vi "Dashboard Main.vi"() -> ()   [LabVIEW 2013]
uses:
  <vilib>/event_ctls.llb/eventvkey.ctl
  <vilib>/Rock Robotics/WPI/Dashboard/WPI_DashboardLogging Global.vi
  <vilib>/Utility/config.llb/Write Key (String).vi
  <vilib>/Utility/config.llb/Write Key (I32).vi
  <vilib>/Utility/config.llb/NI_LVConfig.lvlib
panel:
  out "Camera Image 2":T1(plugin-control)
  out "Image Message":string="Timeout in Camera Communications"
  in  "Rec Mode":enum32{"Stop", "Record", "Playback"}(radio)
  in  "Dashboard Tab":T2(tab)
  in  "Camera Settings":T3={"Frame Rate"=30, "Compression"=30, "Size"=1} {"Frame Rate" scale=1.0..30.0; "Size" items=["640x480", "320x240", "160x120"]}
  out "MotorSliders R":cluster{"MotorSlide1":dbl, "MotorSlide2":dbl} {"MotorSlide2" scale=-1.0..1.0 scale format="%#_2e"; "MotorSlide1" scale=-1.0..1.0 scale format="%#_2e"}
  out "MotorChart R":cluster{"Numeric":dbl, "Numeric":dbl}(graph)
  out "MotorSliders L":T4 {"MotorSlide4 2" scale=0.0..14.0 scale format="%#_2e"; "MotorSlide2" scale=-1.0..1.0 scale format="%#_2e"; "MotorSlide1" scale=-1.0..1.0 scale format="%#_2e"}
  out "MotorChart L":T5(graph)
  out "JS1 Z":dbl(slide) scale=-1.0..1.0 scale format="%#_2e"
  out "Joystick 1":cluster{"X":dbl, "Y":dbl}[](graph)
  out "JS Buttons 1":T6
  out "JS2 Z":dbl(slide) scale=-1.0..1.0 scale format="%#_2e"
  out "Joystick 2":cluster{"X":dbl, "Y":dbl}[](graph)
  out "JS Buttons 2":T6
  out "Mode":T7(ring)=enum."Auto Disabled"
  out "Camera IP":string
  in  "DB Camera Config":bool
  out "fps":dbl format="%#.1g"
  out "Mbps":dbl format="%#.1g"
  out "Mbps 2":bool
  out "LED 1":bool
  out "Pressure":dbl(knob) scale=0.0..120.0
  out "Distance From Wall":dbl(knob) scale=0.0..2.0
  in  "Checkbox 2":bool
  in  "Checkbox 1":bool
  in  "Test Slider":dbl(slide) scale=0.0..100.0 scale format="%#_3g"
  in  "On/Off":bool caption="Solenoid"
  in  "Test Name":u16(ring) items=["Select the test to run...", "Example Test", "-------------------------------", "List of tests is built in robot code.", "Replace with your own automated tests."]
  in  "Test Tree":string(tree)
  in  "Motor":cluster{"Value":dbl, "Enable":bool} {"Value" scale=-1.0..1.0 scale format="%#_3g"}
  out "Progress":T8 {"Test Progress" scale=0.0..100.0}
  in  "Rev/Fwd":cluster{"Forward":bool, "Reverse":bool}
  in  "Test Ring":u16(ring) items=["Auto", "Fixed indoor", "Fixed outdoor 1", "Fixed outdoor 2", "Fixed fluorescent 1", "Fixed fluorescent 2", "Hold current"]
  in  "Listbox":i32(listbox)
  out "Tree":string(tree)
  out "Camera Image":T1(plugin-control)
  in  "Enable":bool
  # "Left"
  # "Front"
  # "Right"
  # "Battery"
  # "Customize by placing controls and indicators here and name to\nmatch Dashboard Variables on robot."
  # "This tab is a great place for autonomous settings and validation.\nCustomize by placing controls and indicators here and name to\nmatch Dashboard Variables on robot."
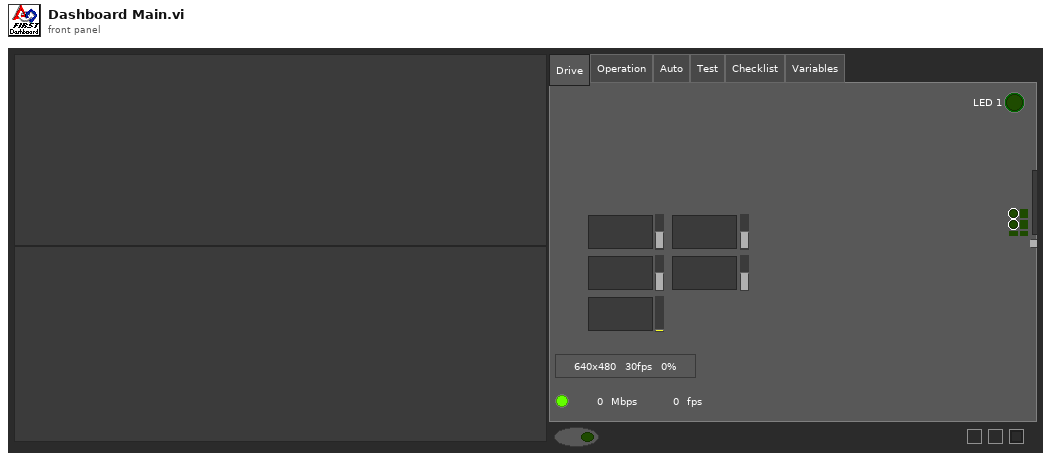
[diagram p1: front panel]
types:
  T1 = typedef "IMAQ Image.ctl" = refnum<image>
  T2 = enum32{"Drive", "Operation", "Auto", "Test", "Checklist", "Variables"}
  T3 = cluster{"Frame Rate":i32, "Compression":i32, "Size":u16}
  T4 = cluster{"MotorSlide1":dbl, "MotorSlide2":dbl, "MotorSlide4 2":dbl}
  T5 = cluster{"Numeric":dbl, "Numeric":dbl, "Battery":sgl}
  T6 = cluster{bool, bool, bool, bool, bool, bool, bool, bool, bool, bool, bool, bool}
  T7 = enum8{"Tele-Op Disabled", "Tele-Op Enabled", "Auto Disabled", "Auto Enabled", "Test Disabled", "Test Enabled", ""}
  T8 = cluster{"Test Progress":u8, "Test Progress Text":string}
  T9 = typedef "Image Type" = u32
  T10 = cluster{"Digital Inputs":bool[], "Digital Outputs":bool[]}
  T11 = cluster{"Competition mode":bool, "Robot Link":bool, "Autonomous":bool, "Enabled":bool, "E-Stop":bool, "Simulated":bool, "TestMode":bool, "Docked Window":bool}
  T12 = cluster{"Boolean Array[0]":bool, "Boolean Array[1]":bool, "Boolean Array[2]":bool, "Boolean Array[3]":bool, "Boolean Array[4]":bool, "Boolean Array[5]":bool, "Boolean Array[6]":bool, "Boolean Array[7]":bool, "Boolean Array[8]":bool, "Boolean Array[9]":bool, "Boolean Array[10]":bool, "Boolean Array[11]":bool}
  T13 = typedef "NI_LVConfig.lvlib/Config Data RefNum.ctl" = refnum<k1>
  T14 = typedef "eventvkey.ctl" = enum16{"ASCII", "Enter", "Return", "Shift", "Ctrl", "Alt", "Cmd", "Opt", "Caps", "NumLock", "Clear", "Break", "Up", "Down", "Left", "Right", "Insert", "Delete", "Home", "End", "PageUp", "PageDown", "Escape", "Help", "Pause", "ScrollLock", "F1", "F2", "F3", "F4", "F5", "F6", "F7", "F8", "F9", "F10", "F11", "F12", "F13", "F14", "F15", "F16", "F17", "F18", "F19", "F20", "F21", "F22", "F23", "F24", "Play", "VolumeUp", "VolumeDown", "Mute", "Two Byte Char"}
  T15 = cluster{"Image Size":bool, "Image Type":bool, "Pixel Value":bool, "ROI Information":bool, "Zoom Factor":bool}
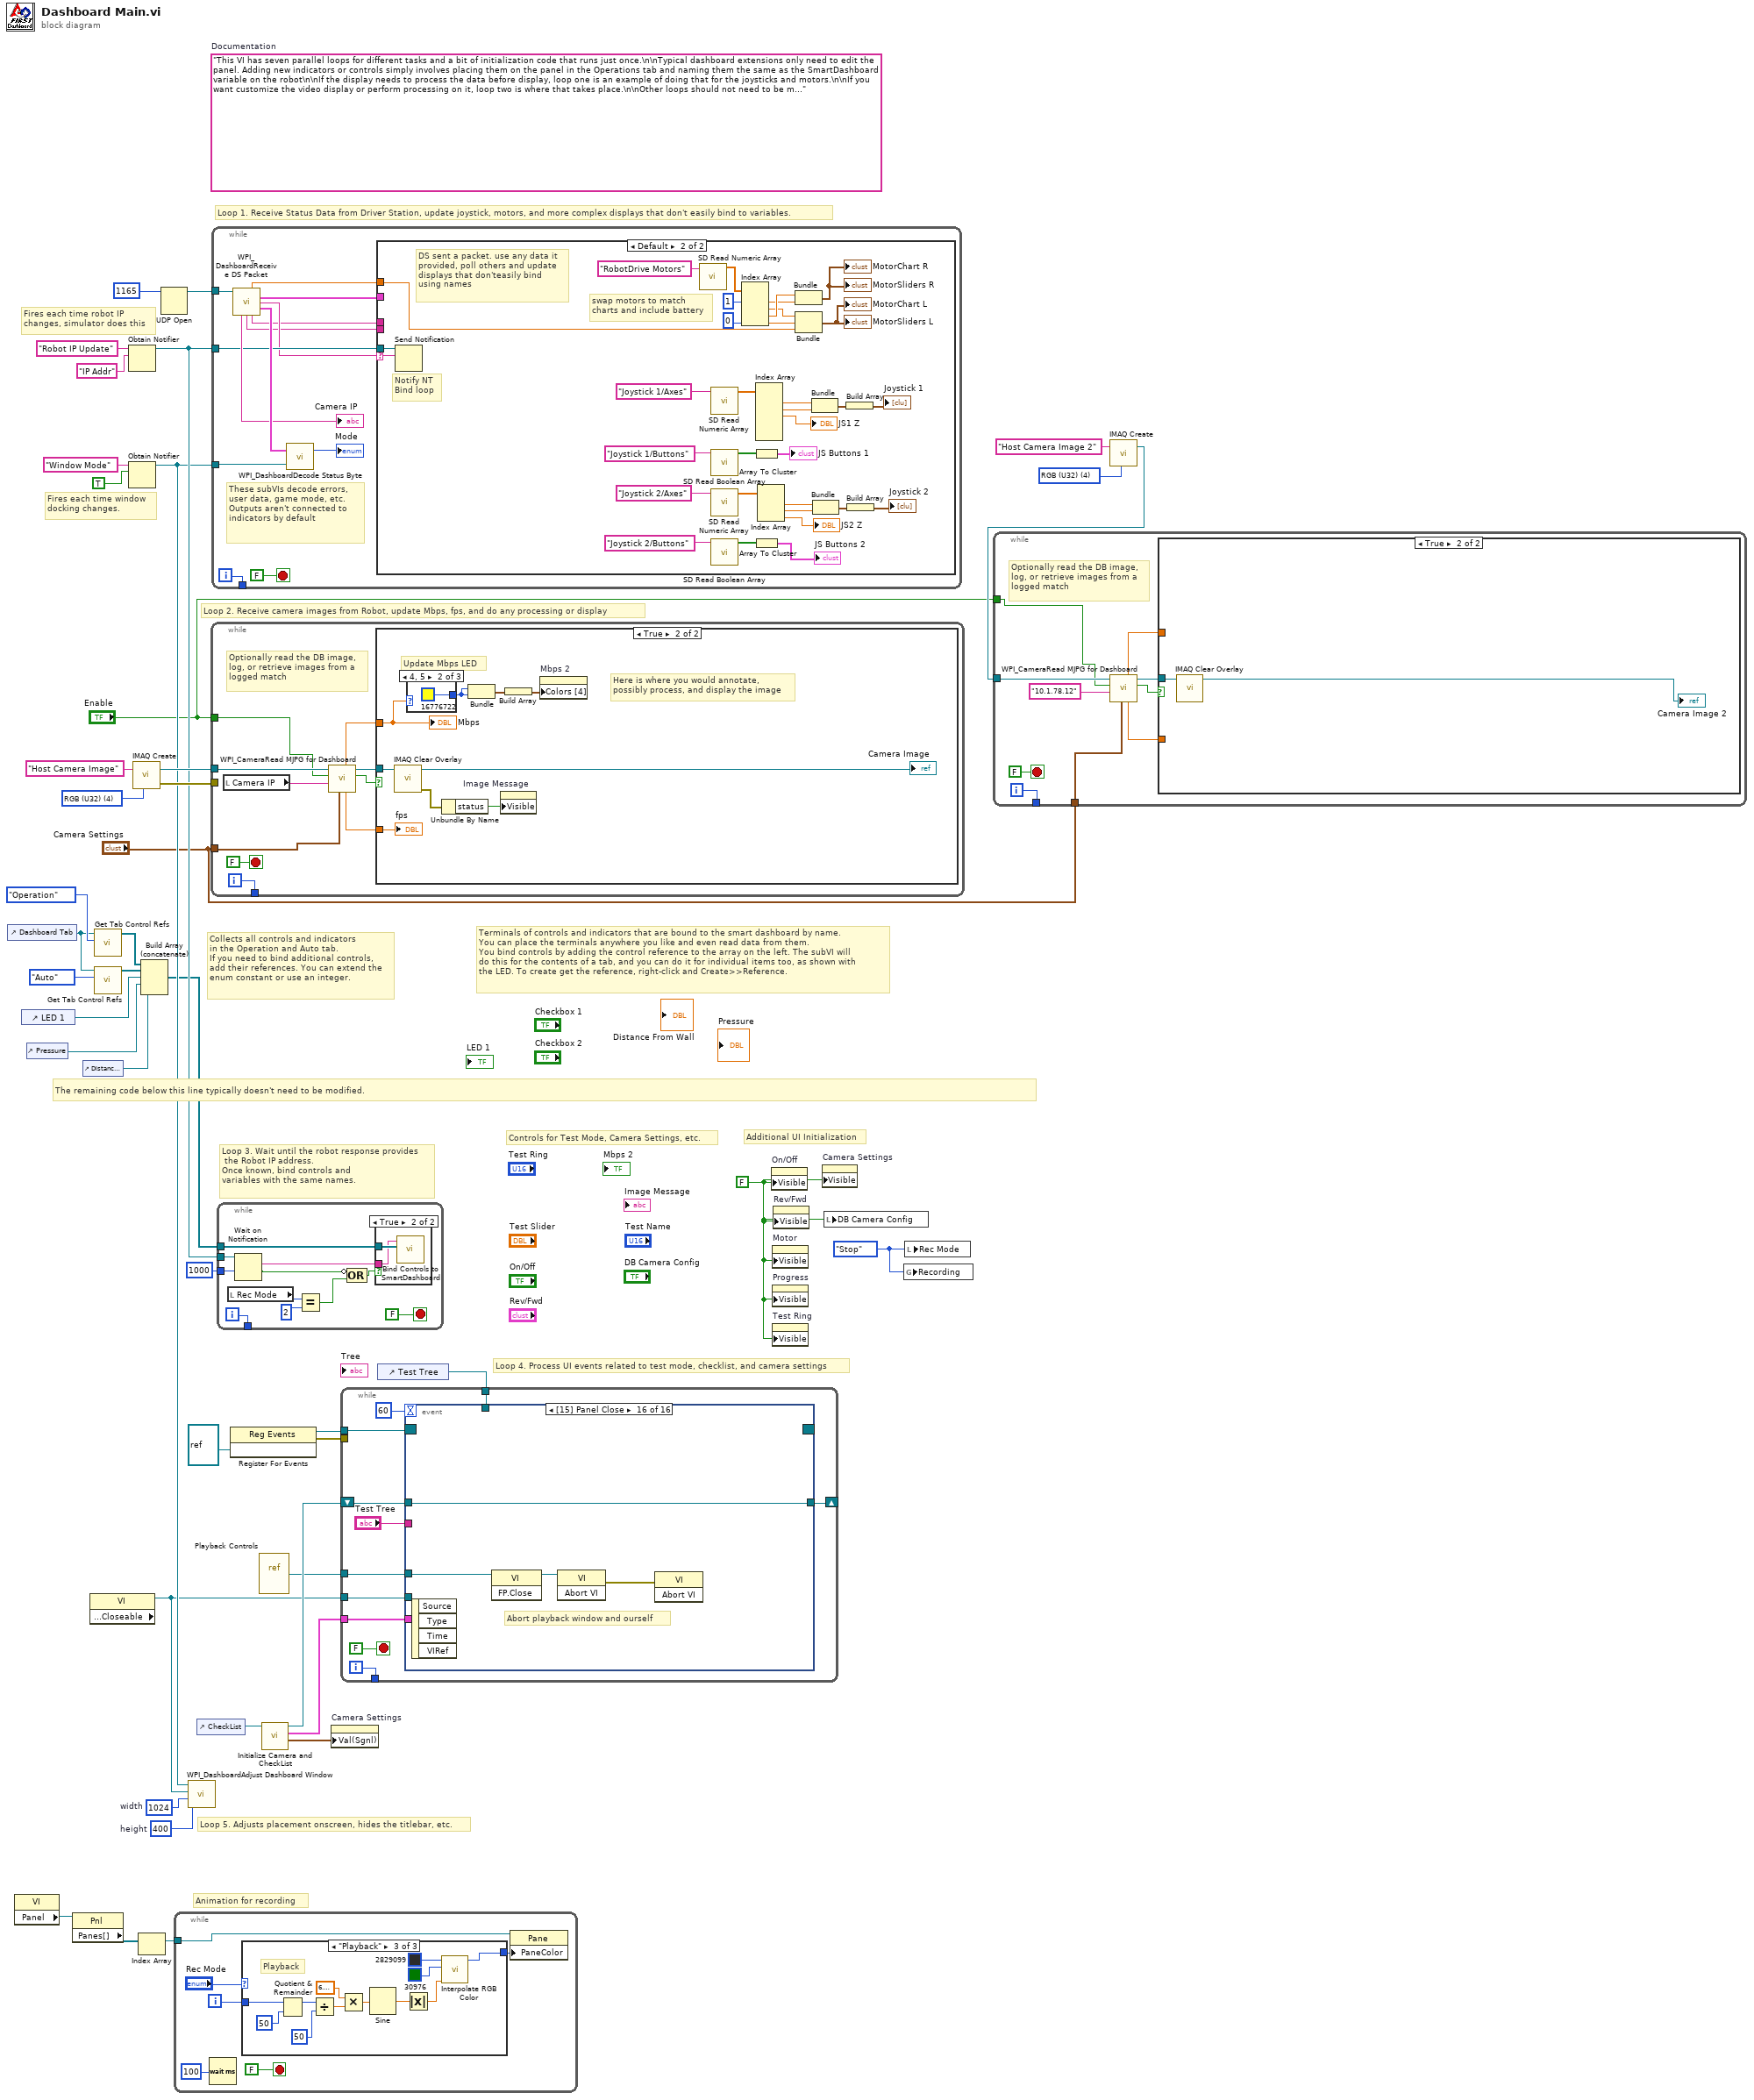
[diagram p0: block diagram]
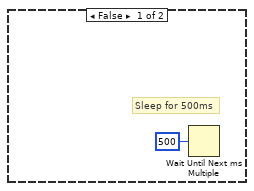
[diagram p2: hidden frame]
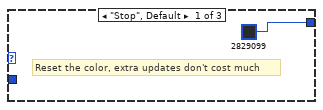
[diagram p3: hidden frame]
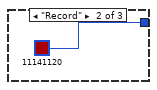
[diagram p4: hidden frame]
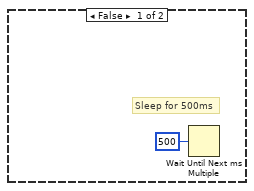
[diagram p6: hidden frame]
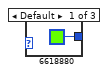
[diagram p7: hidden frame]
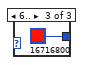
[diagram p8: hidden frame]
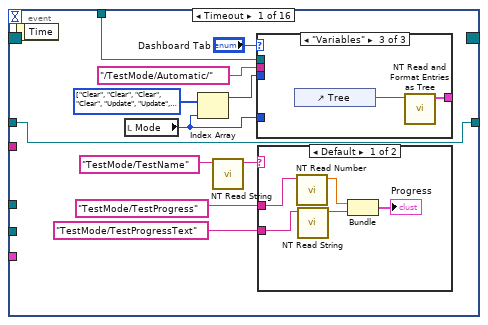
[diagram p9: hidden frame]
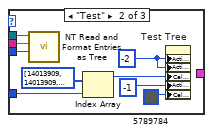
[diagram p11: hidden frame]
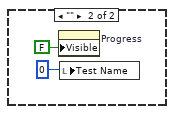
[diagram p12: hidden frame]
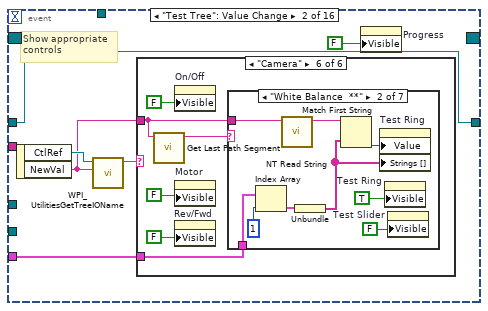
[diagram p13: hidden frame]
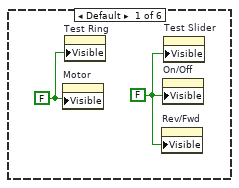
[diagram p14: hidden frame]
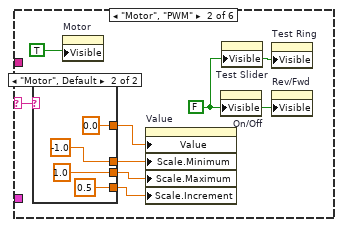
[diagram p15: hidden frame]
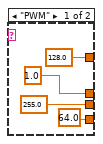
[diagram p16: hidden frame]
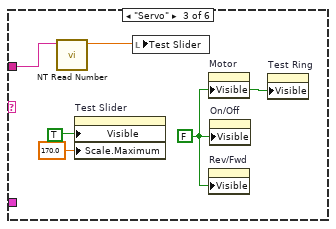
[diagram p17: hidden frame]
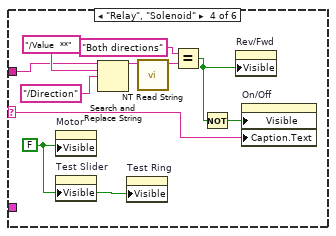
[diagram p18: hidden frame]
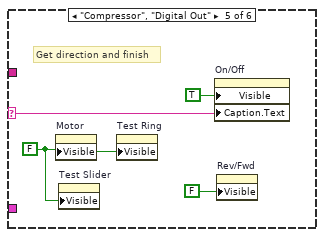
[diagram p19: hidden frame]
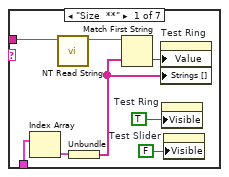
[diagram p20: hidden frame]
diagram:
  w5 = T9 4 items=["Grayscale (U8)", "Grayscale (I16)", "Grayscale (SGL)", "Complex (CSG)", "RGB (U32)", "HSL (U32)", "RGB (U64)"] ("Image Type")
  w15 = enum32{"Stop", "Record", "Playback"}."Stop" ("Rec Mode")
  w18 = 400  # height
  w19 = 1024  # width
  w32 = FALSE ("Visible")
  (unwired) "This VI has seven parallel loops for different tasks and a bit of initialization code that runs just once.\n\nTypical dashboard extensions only need to edit the panel. Adding new indicators or controls simply involves placing them on the panel in the Operations tab and naming them the same as the SmartDashboard variable on the robot\n\nIf the display needs to process the data before display, loop one is an example of doing that for the joysticks and motors.\n\nIf you want customize the video display or perform processing on it, loop two is where that takes place.\n\nOther loops should not need to be modified. They are pretty standard, and document the task they perform."  # Documentation
  w42 = T9 4 items=["Grayscale (U8)", "Grayscale (I16)", "Grayscale (SGL)", "Complex (CSG)", "RGB (U32)", "HSL (U32)", "RGB (U64)"] ("Image Type")
  # "Controls for Test Mode, Camera Settings, etc."
  # "Additional UI Initialization"
  # "Animation for recording"
  # "Fires each time robot IP\nchanges, simulator does this"
  # "Fires each time window\ndocking changes."
  # "Collects all controls and indicators\nin the Operation and Auto tab.\nIf you need to bind additional controls,\nadd their references. You can extend the\nenum constant or use an integer."
  # "The remaining code below this line typically doesn't need to be modified."
  # "Loop 4. Process UI events related to test mode, checklist, and camera settings"
  # "Terminals of controls and indicators that are bound to the smart dashboard by name.\nYou can place the terminals anywhere you like and even read data from them.\nYou bind controls by adding the control reference to the array on the left. The subVI will\ndo this for the contents of a tab, and you can do it for individual items too, as shown with\nthe LED. To create get the reference, right-click and Create>>Reference."
  # "Loop 3. Wait until the robot response provides\n the Robot IP address.\nOnce known, bind controls and\nvariables with the same names."
  # "Loop 5. Adjusts placement onscreen, hides the titlebar, etc."
  # "Loop 1. Receive Status Data from Driver Station, update joystick, motors, and more complex displays that don't easily bind to variables."
  # "Loop 2. Receive camera images from Robot, update Mbps, fps, and do any processing or display"
  n1 = control-ref of="Dashboard Tab"() -> (w13:refnum<vi>)
  n2 = property class="VI"() -> ("Panel"=w26:refnum<vi>)  [unwired: 2 in, 2 out]
  n3 = control-ref of="LED 1"() -> (w8:refnum<vi>)
  n4 = control-ref of="Pressure"() -> (w7:refnum<vi>)
  n5 = property class="Pnl"(reference=w26) -> ("Panes[]"=w27:refnum<vi>[])  [unwired: 1 in, 2 out]
  n6 = control-ref of="Distance From Wall"() -> (w6:refnum<vi>)
  n7 = property class="VI" props=["Front Panel.Closeable"]() -> (reference out=w14:refnum<vi>)  [unwired: 2 in, 2 out]
  n8 = call <vilib>:"Get Tab Control Refs.vi"("Page Index"=T2."Operation" ("Dashboard Tab"), "TabControl in"=w13) -> ("ControlsOnPage"=w11:refnum<vi>[])  [unwired: 9 in]
  n9 = call <vilib>:"Get Tab Control Refs.vi"("Page Index"=T2."Auto" ("Dashboard Tab"), "TabControl in"=w13) -> ("ControlsOnPage"=w12:refnum<vi>[])  [unwired: 9 in]
  n10 = Obtain Notifier(name (unnamed)="Robot IP Update", notification data type="IP Addr" ("name (unnamed)")) -> (notifier out=w36:refnum<notifier>)  [unwired: 2 in, 2 out]
  n11 = Obtain Notifier(name (unnamed)="Window Mode", notification data type=TRUE) -> (notifier out=w17:refnum<notifier>)  [unwired: 2 in, 2 out]
  n12 = call "IMAQ Create"("Image Name"="Host Camera Image", "Image Type"=w42) -> ("New Image"=w40:T1, "error out"=w39:errorcluster)  [unwired: 2 in, 1 out]
  n13 = Index Array(array=w27) -> (element=w25:refnum<vi>)  [unwired: 1 in]
  n14 = Build Array (concatenate)(w11, w12, w8, w7, w6) -> (w10:refnum<vi>[])
  n15 = UDP Open(11:u16 1165 ("port")) -> (port=w43:refnum<k16>)  [unwired: 2 in, 4 out]
  n16 = while {
    tunnel: w25 -> [w46]
    i -> [w49]
    stop <- FALSE stop-if-true
    n17 = Wait (ms)(milliseconds to wait=u32 100) -> ()  [unwired: 1 out]
    n18 = case shown="\"Playback\"" "Rec Mode" {
      tunnel: w49 -> [_ _ w64]
      tunnel: [u32 2829099 ("Base Color") u32 11141120 ("Target Color") w53] -> w45
      frame "Stop", Default {
        # "Reset the color, extra updates don't cost much"
      }
      frame "Record" {
      }
      frame "Playback" {
        # "Playback"
        n19 = Quotient & Remainder(x=w64, y=u32 50 ("milliseconds to wait")) -> (x-y*floor(x/y)=w60:u32)  [unwired: 1 out]
        n20 = Divide(x=w60, y=u32 50 ("milliseconds to wait")) -> (x/y=w57:dbl)
        n21 = Multiply(x=6.283185307179586, y=w57) -> (x*y=w62:dbl)
        n22 = Sine(x=w62) -> (sin(x)=w61:dbl)
        n23 = Absolute Value(x=w61) -> (abs(x)=w54:dbl)
        n24 = call "Interpolate RGB Color.vi"("Proportion"=w54, "Target Color"=u32 30976, "Base Color"=u32 2829099) -> ("Result Color"=w53:u32)  [unwired: 8 in]
      }
    }
    n25 = property class="Pane"(reference=w46, "PaneColor"=w45) -> ()  [unwired: 1 in, 2 out]
  }
  n26 = call <vilib>:"WPI_DashboardAdjust Dashboard Window.vi"("height"=w18, "width"=w19, "reference in"=w14, "Notifier in"=w17) -> ()  [unwired: 8 in]
  n27 = control-ref of="CheckList"() -> (w16:refnum<vi>)
  n28 = while {
    tunnel: w40 -> [w72]
    tunnel: w39 -> [_]
    tunnel: [w73] -> _
    tunnel: "Camera Settings" -> [w66]
    tunnel: "Enable" -> [w65]
    i -> [w73]
    stop <- FALSE stop-if-true
    # "Optionally read the DB image,\nlog, or retrieve images from a\nlogged match"
    n29 = local read "Camera IP"() -> (w67:string)
    n30 = call <vilib>:"WPI_CameraRead MJPG for Dashboard.vi"("Camera Settings"=w66, "Camera IP"=w67, "Enable"=w65, "Refnum in"=w72) -> ("Active"=w70:bool, "Refnum out"=w71:T1, "FPS"=w69:dbl, "Bandwidth (Mbps)"=w68:dbl)  [unwired: 4 in]
    n31 = case shown="True" w70 {
      tunnel: w71 -> [_ w79]
      tunnel: w68 -> [_ w78]
      tunnel: w69 -> [_ w76]
      frame False {
        # "Sleep for 500ms"
        n32 = Wait Until Next ms Multiple(millisecond multiple=u32 500) -> ()  [unwired: 1 out]
      }
      frame True {
        # "Here is where you would annotate,\npossibly process, and display the image"
        # "Update Mbps LED"
        n33 = call "IMAQ Clear Overlay"("Image"=w79) -> ("error out"=w83:errorcluster, "Image Out"=→"Camera Image":T1)  [unwired: 2 in, 7 out]
        n34 = case shown="4, 5" w78 {
          tunnel: [u32 6618880 ("Color Box") u32 16776722 ("Color Box") u32 16716800 ("Color Box")] -> w80
          frame Default {
          }
          frame 4, 5 {
          }
          frame 6.. {
          }
        }
        n35 = Unbundle By Name(w83) -> ("status"=w84:bool)
        n36 = Bundle("Color Box"=w80, "Color Box"=w80) -> (w82:cluster{"Color Box":u32, "Color Box":u32})  [unwired: 1 out]
        n37 = property on="Image Message" class="Str"("Visible"=w84) -> ()  [unwired: 2 in, 2 out]
        n38 = Build Array(w82) -> (w81:cluster{"Color Box":u32, "Color Box":u32}[])
        n39 = property on="Mbps 2" class="Bool (strict)"("Colors [4]"=w81) -> ()  [unwired: 2 in, 2 out]
        "Mbps" <- w78
        "fps" <- w76
      }
    }
  }
  n40 = while {
    tunnel: w43 -> [w98]
    tunnel: w36 -> [w93]
    tunnel: w17 -> [w97]
    tunnel: [w94] -> _
    i -> [w94]
    stop <- FALSE stop-if-true
    # "These subVIs decode errors, user data, game mode, etc.\nOutputs aren't connected to indicators by default"
    n41 = call <vilib>:"WPI_DashboardReceive DS Packet.vi"("Recv Socket"=w98) -> ("Battery"=w88:sgl, "Driver Station"=w89:T10, "Robot IP Address"=w92:string, "Status"=w99:T11, "Camera IP Address"=→"Camera IP":string, "Low Priority User Data"=w91:string, "High Priority User Data"=w90:string)  [unwired: 1 in, 7 out]
    n42 = call <vilib>:"WPI_DashboardDecode Status Byte.vi"("Window Mode Notifier"=w97, "Status"=w99) -> ("Mode"=→"Mode":T7)  [unwired: 1 out]
    n43 = case shown="Default" w92 {
      selector: w92 -> [_ w111]
      tunnel: w93 -> [_ w112]
      tunnel: w91 -> [_ _]
      tunnel: w90 -> [_ _]
      tunnel: w89 -> [_ _]
      tunnel: w88 -> [_ w110]
      frame "0.0.0.0" {
        # "DS not sending packets, or no robot exists yet.\nDon't poll the variables"
      }
      frame Default {
        # "Notify NT\nBind loop"
        # "DS sent a packet. use any data it\nprovided, poll others and update\ndisplays that don'teasily bind\nusing names"
        # "swap motors to match\ncharts and include battery"
        n44 = Send Notification(notification=w111, notifier=w112) -> ()  [unwired: 1 in, 2 out]
        n45 = call <vilib>:"SD Read Numeric Array.vi"("Name"="RobotDrive Motors") -> ("Numeric Array"=w109:dbl[])  [unwired: 8 in, 2 out]
        n46 = call <vilib>:"SD Read Numeric Array.vi"("Name"="Joystick 1/Axes") -> ("Numeric Array"=w128:dbl[])  [unwired: 8 in, 2 out]
        n47 = call <vilib>:"SD Read Boolean Array.vi"("Name"="Joystick 1/Buttons") -> ("Boolean Array"=w130:bool[])  [unwired: 8 in, 2 out]
        n48 = call <vilib>:"SD Read Numeric Array.vi"("Name"="Joystick 2/Axes") -> ("Numeric Array"=w122:dbl[])  [unwired: 8 in, 2 out]
        n49 = call <vilib>:"SD Read Boolean Array.vi"("Name"="Joystick 2/Buttons") -> ("Boolean Array"=w121:bool[])  [unwired: 8 in, 2 out]
        n50 = Index Array(array=w109, index #1=1, index #4=0) -> (element #1=w105:dbl, element #2=w104:dbl, element #3=w106:dbl, element #4=w101:dbl)  [unwired: 2 in]
        n51 = Array To Cluster(array=w130) -> (cluster=→"JS Buttons 1":T12)
        n52 = Array To Cluster(array=w121) -> (cluster=→"JS Buttons 2":T12)
        n53 = Index Array(array=w128) -> (element #1=w125:dbl, element #2=w126:dbl, element #3=→"JS1 Z":dbl)  [unwired: 6 in, 3 out]
        n54 = Index Array(array=w122) -> (element #1=w117:dbl, element #2=w116:dbl, element #3=→"JS2 Z":dbl)  [unwired: 3 in]
        n55 = Bundle("Numeric"=w106, "Numeric"=w105) -> (→"MotorChart R" →"MotorSliders R":cluster{"Numeric":dbl, "Numeric":dbl})  [unwired: 1 in]
        n56 = Bundle("Numeric"=w104, "Numeric"=w101, "Battery"=w110) -> (→"MotorChart L" →"MotorSliders L":T5)  [unwired: 1 in]
        n57 = Bundle("Numeric"=w125, "Numeric"=w126) -> (w124:cluster{"Numeric":dbl, "Numeric":dbl})  [unwired: 1 in]
        n58 = Bundle("Numeric"=w117, "Numeric"=w116) -> (w118:cluster{"Numeric":dbl, "Numeric":dbl})  [unwired: 1 in]
        n59 = Build Array(w124) -> (→"Joystick 1":cluster{"Numeric":dbl, "Numeric":dbl}[])
        n60 = Build Array(w118) -> (→"Joystick 2":cluster{"Numeric":dbl, "Numeric":dbl}[])
      }
    }
  }
  n61 = while {
    tunnel: w10 -> [w144]
    tunnel: w36 -> [w142]
    tunnel: [w140] -> _
    tunnel: u32 1000 ("milliseconds to wait") -> [w139]
    i -> [w140]
    stop <- FALSE stop-if-true
    n62 = local read "Rec Mode"() -> (w135:enum32{"Stop", "Record", "Playback"})
    n63 = Wait on Notification(notifier=w142, timeout in ms (-1)=w139) -> (notification=w141:string, timed out?=w137:bool)  [unwired: 2 in, 2 out]
    n64 = Equal?(x=w135, y=u16 2 ("Rec Mode")) -> (x = y?=w136:bool)
    n65 = Compound Arithmetic op=OR(invert w137, w136) -> (w138:bool)
    n66 = case shown="True" w138 {
      tunnel: w144 -> [_ w146]
      tunnel: w141 -> [_ w145]
      frame False {
      }
      frame True {
        n67 = call <vilib>:"Bind Controls to SmartDashboard.vi"("Bound Control Refs"=w146, "Server IP Address"=w145) -> ()  [unwired: 10 in]
      }
    }
  }
  n68 = register-events(refnum<vi> refnum) -> (reference out=w23:refnum<event-registration>, error out=w22:errorcluster)  [unwired: 2 in]
  n69 = vi-ref "Playback Controls.vi"() -> (w24:refnum<vi>)
  n70 = call "Initialize Camera and CheckList.vi"("ListBox in"=w16) -> ("Cluster"=w30:cluster{"value":i32, "value":i32, "index":i32}, "Array"=w31:cluster{string[]}[], "File Refnum"=w29:T13)  [unwired: 8 in]
  n71 = property on="Camera Settings" class="Clust (strict)"("Val(Sgnl)"=w30) -> ()  [unwired: 2 in, 2 out]
  n72 = control-ref of="Test Tree"() -> (w28:refnum<vi>)
  n73 = while {
    tunnel: w31 -> [w154]
    shift-right: [w153] -> _
    shift-left: w29 -> [w152]
    tunnel: [w151] -> _
    tunnel: w28 -> [w150]
    tunnel: w24 -> [w149]
    tunnel: w23 -> [w148]
    tunnel: w22 -> [_]
    tunnel: w14 -> [w147]
    i -> [w151]
    stop <- FALSE stop-if-true
    n74 = event shown="[15] Panel Close" {
      selector: w148 -> [_ _ _ _ _ _ _ _ _ _ _ _ _ _ _ _]
      dyn-events: [_ _ _ _ _ _ _ _ _ _ _ _ _ w392 _ _] -> _
      timeout: u32 60 ("milliseconds to wait") -> [_ _ _ _ _ _ _ _ _ _ _ _ _ _ _ _]
      tunnel: w150 -> [w164 _ _ _ _ _ _ _ _ _ _ _ _ _ _ _]
      tunnel: "Test Tree" -> [_ _ _ _ _ _ _ _ w361 w369 w371 w375 w383 _ _ _]
      tunnel: w154 -> [_ w188 _ _ _ _ w325 w355 _ _ _ _ _ _ _ _]
      tunnel: [w158 w187 w286 w291 w299 w311 w324 w348 w360 w367 w370 w374 w382 w394 w408 w409] -> w153
      tunnel: w152 -> [w158 w187 w286 w291 w299 w311 w323 w348 w360 w367 w370 w374 w382 w394 w408 w409]
      tunnel: w149 -> [_ _ _ _ _ _ _ _ _ _ _ _ _ w395 _ w412]
      tunnel: w147 -> [_ _ _ _ _ _ _ _ _ _ _ _ _ w390 _ _]
      event Timeout {
        w163 = enum16{"Update", "Clear"}[] [enum."Clear", enum."Clear", enum."Clear", enum."Clear", enum."Update", enum."Update", enum."Clear"] items=["Update", "Clear"]
        n75 = event-data() -> ()  [unwired: 1 in, 1 out]
        n76 = local read "Mode"() -> (w161:T7)
        n77 = Index Array(array=w163, index=w161) -> (element=w162:enum16{"Update", "Clear"})
        n78 = call <vilib>:"NT Read String.vi"("Name"="TestMode/TestName") -> ("String"=w167:string)  [unwired: 9 in, 1 out]
        n79 = case shown="\"Variables\"" "Dashboard Tab" {
          tunnel: w164 -> [_ w177 _]
          tunnel: "/TestMode/Automatic/" ("Name Pattern") -> [_ w176 _]
          tunnel: w162 -> [_ w175 _]
          tunnel: w161 -> [_ w173 _]
          tunnel: [_ _ w179] -> _
          frame "Operation", Default {
          }
          frame "Test" {
            w172 = -2 ("Active Item:Row Number")
            n80 = call <vilib>:"NT Read and Format Entries as Tree.vi"("Operation"=w175, "Name Pattern"=w176, "Tree Refnum"=w177) -> ()  [unwired: 7 in, 2 out]
            n81 = Index Array(array=u32[] [14013909, 14013909, 14013909, 14013909, 14013909, 16777215, 14013909], index=w173) -> (element=w171:u32)
            n82 = property on="Test Tree" class="Tree (strict)"("Active Item Row Number"=w172, "ActiveColNum"=w172, "CellBG"=w171, "Active Item Row Number"=-1 ("Active Item:Row Number"), "CellBG"=u32 5789784 ("Color Box")) -> ()  [unwired: 2 in, 2 out]
          }
          frame "Variables" {
            n83 = control-ref of="Tree"() -> (w178:refnum<vi>)
            n84 = call <vilib>:"NT Read and Format Entries as Tree.vi"("Tree Refnum"=w178) -> ("Formatted Strings"=w179:cluster{"Name":string, "Value":string}[])  [unwired: 9 in, 1 out]
          }
        }
        n85 = case shown="Default" w167 {
          tunnel: "TestMode/TestProgress" ("Name") -> [w181 _]
          tunnel: "TestMode/TestProgressText" ("Name") -> [w180 _]
          frame Default {
            n86 = call <vilib>:"NT Read Number.vi"("Name"=w181) -> ("Numeric"=w182:dbl)  [unwired: 9 in, 1 out]
            n87 = call <vilib>:"NT Read String.vi"("Name"=w180) -> ("String"=w183:string)  [unwired: 9 in, 1 out]
            n88 = Bundle("Numeric"=w182, "String"=w183) -> (→"Progress":cluster{"Numeric":dbl, "String":string})  [unwired: 1 in]
          }
          frame "" {
            n89 = property on="Progress" class="Clust (strict)"("Visible"=FALSE) -> ()  [unwired: 2 in, 2 out]
            n90 = local write "Test Name"(u16 0) -> ()
          }
        }
      }
      event "Test Tree": Value Change {
        # "Show appropriate\ncontrols"
        n91 = event-data() -> ("CtlRef"=w191:refnum<vi>, "NewVal"=w189:string)  [unwired: 1 in]
        n92 = call <vilib>:"WPI_UtilitiesGetTreeIOName.vi"("NewVal"=w189, "TreeControl in"=w191) -> ("I/O Name"=w192:string)  [unwired: 9 in]
        n93 = case shown="\"Camera\"" w192 {
          selector: w192 -> [_ w199 _ w217 w226 _]
          tunnel: w189 -> [_ _ w214 w216 _ w233]
          tunnel: w188 -> [_ _ _ _ _ w232]
          frame Default {
            w194 = FALSE ("Visible")
            w193 = FALSE ("Visible")
            n94 = property on="Motor" class="Clust (strict)"("Visible"=w193) -> ()  [unwired: 2 in, 2 out]
            n95 = property on="Test Ring" class="Ring (strict)"("Visible"=w193) -> ()  [unwired: 2 in, 2 out]
            n96 = property on="Rev/Fwd" class="Clust (strict)"("Visible"=w194) -> ()  [unwired: 2 in, 2 out]
            n97 = property on="On/Off" class="Bool (strict)"("Visible"=w194) -> ()  [unwired: 2 in, 2 out]
            n98 = property on="Test Slider" class="Slide (strict)"("Visible"=w194) -> ()  [unwired: 2 in, 2 out]
          }
          frame "Motor", "PWM" {
            w200 = FALSE ("Visible")
            n99 = case shown="\"Motor\", Default" w199 {
              tunnel: [1.0 ("Value") -1.0 ("Value")] -> w198
              tunnel: [255.0 ("Value") 1.0 ("Value")] -> w197
              tunnel: [128.0 ("Value") 0.0 ("Value")] -> w196
              tunnel: [64.0 ("Value") 0.5 ("Value")] -> w195
              frame "PWM" {
              }
              frame "Motor", Default {
              }
            }
            n100 = property on="Motor" class="Clust (strict)"("Visible"=TRUE) -> ()  [unwired: 2 in, 2 out]
            n101 = property on="Value" class="Slide (strict)"("Value"=w196, "Scale.Minimum"=w198, "Scale.Maximum"=w197, "Scale.Increment"=w195) -> ()  [unwired: 2 in, 2 out]
            n102 = property on="On/Off" class="Bool (strict)"("Visible"=w200) -> ()  [unwired: 2 in, 2 out]
            n103 = property on="Test Slider" class="Slide (strict)"("Visible"=w200) -> ()  [unwired: 2 in, 2 out]
            n104 = property on="Test Ring" class="Ring (strict)"("Visible"=w200) -> ()  [unwired: 2 in, 2 out]
            n105 = property on="Rev/Fwd" class="Clust (strict)"("Visible"=w200) -> ()  [unwired: 2 in, 2 out]
          }
          frame "Servo" {
            w212 = FALSE ("Visible")
            n106 = call <vilib>:"NT Read Number.vi"("Name"=w214) -> ("Numeric"=w213:dbl)  [unwired: 9 in, 1 out]
            n107 = property on="Test Slider" class="Slide (strict)"("Visible"=TRUE, "Scale.Maximum"=170.0 ("Scale.Range:Maximum")) -> ()  [unwired: 2 in, 2 out]
            n108 = local write "Test Slider"(w213) -> ()
            n109 = property on="Motor" class="Clust (strict)"("Visible"=w212) -> ()  [unwired: 2 in, 2 out]
            n110 = property on="Rev/Fwd" class="Clust (strict)"("Visible"=w212) -> ()  [unwired: 2 in, 2 out]
            n111 = property on="On/Off" class="Bool (strict)"("Visible"=w212) -> ()  [unwired: 2 in, 2 out]
            n112 = property on="Test Ring" class="Ring (strict)"("Visible"=w212) -> ()  [unwired: 2 in, 2 out]
          }
          frame "Relay", "Solenoid" {
            w215 = FALSE ("Visible")
            n113 = property on="Motor" class="Clust (strict)"("Visible"=w215) -> ()  [unwired: 2 in, 2 out]
            n114 = property on="Test Slider" class="Slide (strict)"("Visible"=w215) -> ()  [unwired: 2 in, 2 out]
            n115 = Search and Replace String(input string=w216, search string="/Value  **", replace string="/Direction") -> (result string=w222:string)  [unwired: 5 in, 3 out]
            n116 = property on="Test Ring" class="Ring (strict)"("Visible"=w215) -> ()  [unwired: 2 in, 2 out]
            n117 = call <vilib>:"NT Read String.vi"("Name"=w222) -> ("String"=w220:string)  [unwired: 9 in, 1 out]
            n118 = Equal?(x="Both directions", y=w220) -> (x = y?=w218:bool)
            n119 = Not(x=w218) -> (.not. x?=w219:bool)
            n120 = property on="Rev/Fwd" class="Clust (strict)"("Visible"=w218) -> ()  [unwired: 2 in, 2 out]
            n121 = property on="On/Off" class="Bool (strict)"("Visible"=w219, "Caption.Text"=w217) -> ()  [unwired: 2 in, 2 out]
          }
          frame "Compressor", "Digital Out" {
            w225 = FALSE ("Visible")
            # "Get direction and finish"
            n122 = property on="Motor" class="Clust (strict)"("Visible"=w225) -> ()  [unwired: 2 in, 2 out]
            n123 = property on="Test Slider" class="Slide (strict)"("Visible"=w225) -> ()  [unwired: 2 in, 2 out]
            n124 = property on="Test Ring" class="Ring (strict)"("Visible"=w225) -> ()  [unwired: 2 in, 2 out]
            n125 = property on="On/Off" class="Bool (strict)"("Visible"=TRUE, "Caption.Text"=w226) -> ()  [unwired: 2 in, 2 out]
            n126 = property on="Rev/Fwd" class="Clust (strict)"("Visible"=FALSE) -> ()  [unwired: 2 in, 2 out]
          }
          frame "Camera" {
            n127 = call <vilib>:"Get Last Path Segment.vi"("String in"=w233) -> ("String out"=w234:string)  [unwired: 10 in]
            n128 = property on="On/Off" class="Bool (strict)"("Visible"=FALSE) -> ()  [unwired: 2 in, 2 out]
            n129 = property on="Motor" class="Clust (strict)"("Visible"=FALSE) -> ()  [unwired: 2 in, 2 out]
            n130 = property on="Rev/Fwd" class="Clust (strict)"("Visible"=FALSE) -> ()  [unwired: 2 in, 2 out]
            n131 = case shown="\"White Balance  **\"" w234 {
              tunnel: w233 -> [w240 w249 w258 w267 w276 _ w282]
              tunnel: w232 -> [w238 w246 w255 w264 w273 _ _]
              frame "Size  **" {
                n132 = Index Array(array=w238) -> (element=w237:cluster{string[]})  [unwired: 1 in]
                n133 = call <vilib>:"NT Read String.vi"("Name"=w240) -> ("String"=w239:string)  [unwired: 9 in, 1 out]
                n134 = Unbundle(w237) -> (w235:string[])
                n135 = Match First String(2:w235, 3:w239) -> (0:w236:i32)  [unwired: 1 out]
                n136 = property on="Test Ring" class="Ring (strict)"("Value"=w236, "Strings []"=w235) -> ()  [unwired: 2 in, 2 out]
                n137 = property on="Test Ring" class="Ring (strict)"("Visible"=TRUE) -> ()  [unwired: 2 in, 2 out]
                n138 = property on="Test Slider" class="Slide (strict)"("Visible"=FALSE) -> ()  [unwired: 2 in, 2 out]
              }
              frame "White Balance  **" {
                n139 = Index Array(array=w246, index=1) -> (element=w247:cluster{string[]})
                n140 = call <vilib>:"NT Read String.vi"("Name"=w249) -> ("String"=w248:string)  [unwired: 9 in, 1 out]
                n141 = Unbundle(w247) -> (w244:string[])
                n142 = Match First String(2:w244, 3:w248) -> (0:w243:i32)  [unwired: 1 out]
                n143 = property on="Test Ring" class="Ring (strict)"("Value"=w243, "Strings []"=w244) -> ()  [unwired: 2 in, 2 out]
                n144 = property on="Test Ring" class="Ring (strict)"("Visible"=TRUE) -> ()  [unwired: 2 in, 2 out]
                n145 = property on="Test Slider" class="Slide (strict)"("Visible"=FALSE) -> ()  [unwired: 2 in, 2 out]
              }
              frame "Exposure  **" {
                n146 = Index Array(array=w255, index=2) -> (element=w256:cluster{string[]})
                n147 = call <vilib>:"NT Read String.vi"("Name"=w258) -> ("String"=w257:string)  [unwired: 9 in, 1 out]
                n148 = Unbundle(w256) -> (w252:string[])
                n149 = Match First String(2:w252, 3:w257) -> (0:w253:i32)  [unwired: 1 out]
                n150 = property on="Test Ring" class="Ring (strict)"("Value"=w253, "Strings []"=w252) -> ()  [unwired: 2 in, 2 out]
                n151 = property on="Test Ring" class="Ring (strict)"("Visible"=TRUE) -> ()  [unwired: 2 in, 2 out]
                n152 = property on="Test Slider" class="Slide (strict)"("Visible"=FALSE) -> ()  [unwired: 2 in, 2 out]
              }
              frame "Exposure Priority  **" {
                n153 = Index Array(array=w264, index=3) -> (element=w265:cluster{string[]})
                n154 = call <vilib>:"NT Read String.vi"("Name"=w267) -> ("String"=w266:string)  [unwired: 9 in, 1 out]
                n155 = Unbundle(w265) -> (w261:string[])
                n156 = Match First String(2:w261, 3:w266) -> (0:w262:i32)  [unwired: 1 out]
                n157 = property on="Test Ring" class="Ring (strict)"("Value"=w262, "Strings []"=w261) -> ()  [unwired: 2 in, 2 out]
                n158 = property on="Test Ring" class="Ring (strict)"("Visible"=TRUE) -> ()  [unwired: 2 in, 2 out]
                n159 = property on="Test Slider" class="Slide (strict)"("Visible"=FALSE) -> ()  [unwired: 2 in, 2 out]
              }
              frame "Color Enable  **" {
                n160 = Index Array(array=w273, index=4) -> (element=w274:cluster{string[]})
                n161 = call <vilib>:"NT Read String.vi"("Name"=w276) -> ("String"=w275:string)  [unwired: 9 in, 1 out]
                n162 = Unbundle(w274) -> (w270:string[])
                n163 = Match First String(2:w270, 3:w275) -> (0:w271:i32)  [unwired: 1 out]
                n164 = property on="Test Ring" class="Ring (strict)"("Value"=w271, "Strings []"=w270) -> ()  [unwired: 2 in, 2 out]
                n165 = property on="Test Ring" class="Ring (strict)"("Visible"=TRUE) -> ()  [unwired: 2 in, 2 out]
                n166 = property on="Test Slider" class="Slide (strict)"("Visible"=FALSE) -> ()  [unwired: 2 in, 2 out]
              }
              frame Default {
                n167 = property on="Test Ring" class="Ring (strict)"("Visible"=FALSE) -> ()  [unwired: 2 in, 2 out]
                n168 = property on="Test Slider" class="Slide (strict)"("Visible"=FALSE) -> ()  [unwired: 2 in, 2 out]
              }
              frame "Brightness  **", "Color Level  **", "Compression  **", "FPS  **", "Sharpness  **" {
                n169 = call <vilib>:"NT Read Number.vi"("Name"=w282) -> ("Numeric"=w281:dbl)  [unwired: 9 in, 1 out]
                n170 = local write "Test Slider"(w281) -> ()
                n171 = property on="Test Slider" class="Slide (strict)"("Visible"=TRUE, "Scale.Maximum"=100.0 ("Scale.Range:Maximum")) -> ()  [unwired: 2 in, 2 out]
                n172 = property on="Test Ring" class="Ring (strict)"("Visible"=FALSE) -> ()  [unwired: 2 in, 2 out]
              }
            }
          }
        }
        n173 = property on="Progress" class="Clust (strict)"("Visible"=FALSE) -> ()  [unwired: 2 in, 2 out]
      }
      event "Test Name": Mouse Enter {
        # "Populate the ring with the list of tests"
        n174 = event-data() -> ()  [unwired: 1 in, 1 out]
        n175 = call <vilib>:"NT Read String Array.vi"("Name"="TestMode/TestList") -> ("String Array"=w290:string[])  [unwired: 9 in, 1 out]
        n176 = Build Array (concatenate)("Select the test to run...", w290) -> (w289:string[])
        n177 = property on="Test Name" class="Ring (strict)"("Strings []"=w289) -> ()  [unwired: 2 in, 2 out]
      }
      event "Test Name": Value Change {
        w292 = FALSE ("Visible")
        # "Tell the robot the test name to run"
        n178 = event-data() -> ("NewVal"=w296:u16)  [unwired: 1 in]
        n179 = property on="Test Name" class="Ring (strict)"() -> ("Strings []"=w297:string[])  [unwired: 2 in, 2 out]
        n180 = local write "Progress"(T8 {"Test Progress"=0, "Test Progress Text"=""} ("Progress")) -> ()
        n181 = Index Array(array=w297, index=w296) -> (element=w295:string)
        n182 = call <vilib>:"NT Write String.vi"("String"=w295, "Name"="TestMode/TestName") -> ()  [unwired: 9 in, 1 out]
        n183 = property on="Progress" class="Clust (strict)"("Visible"=TRUE) -> ()  [unwired: 2 in, 2 out]
        n184 = property on="Motor" class="Clust (strict)"("Visible"=w292) -> ()  [unwired: 2 in, 2 out]
        n185 = property on="Test Slider" class="Slide (strict)"("Visible"=w292) -> ()  [unwired: 2 in, 2 out]
        n186 = property on="On/Off" class="Bool (strict)"("Visible"=w292) -> ()  [unwired: 2 in, 2 out]
        n187 = property on="Rev/Fwd" class="Clust (strict)"("Visible"=w292) -> ()  [unwired: 2 in, 2 out]
        n188 = property on="Test Ring" class="Ring (strict)"("Visible"=w292) -> ()  [unwired: 2 in, 2 out]
      }
      event "Listbox": Double Click {
        n189 = event-data() -> ("PlatMods.Shift"=w300:bool, "Row"=w302:i32)  [unwired: 1 in]
        n190 = case shown="True" w300 {
          tunnel: w302 -> [w306 _]
          tunnel: 1 -> [w305 _]
          frame False {
            n191 = property on="Listbox" class="LstBox (strict)"() -> ("Item Symbols"=w304:i32[])  [unwired: 2 in, 2 out]
            n192 = Replace Array Subset(array=w304, new element=w305, index=w306) -> (w303:i32[])
            n193 = property on="Listbox" class="LstBox (strict)"("Item Symbols"=w303) -> ()  [unwired: 2 in, 2 out]
          }
          frame True {
            w307 = 0 ("Top Row")
            n194 = property on="Listbox" class="LstBox (strict)"() -> ("Number of Rows"=w309:u32)  [unwired: 2 in, 2 out]
            n195 = Initialize Array(0, w309) -> (w308:i32[])
            n196 = property on="Listbox" class="LstBox (strict)"("Top Row"=w307, "Value"=w307, "Item Symbols"=w308) -> ()  [unwired: 2 in, 2 out]
          }
        }
      }
      event "Listbox": Key Down {
        n197 = event-data() -> ("VKey"=w313:T14)  [unwired: 1 in]
        n198 = case shown="\"Left\", \"Right\"" w313 {
          selector: w313 -> [w318 _]
          tunnel: eventvkey."Left" ("VKey") -> [w316 _]
          frame "Left", "Right" {
            n199 = Equal?(x=w316, y=w318) -> (x = y?=w317:bool)
            n200 = Select(t=0, s=w317, f=1) -> (s? t:f=w319:i32)
            n201 = property on="Listbox" class="LstBox (strict)"() -> ("Item Symbols"=w322:i32[])  [unwired: 2 in, 2 out]
            n202 = Replace Array Subset(array=w322, new element=w319, index="Listbox") -> (w321:i32[])
            n203 = property on="Listbox" class="LstBox (strict)"("Item Symbols"=w321) -> ()  [unwired: 2 in, 2 out]
          }
          frame Default {
          }
        }
      }
      event "DB Camera Config": Value Change {
        n204 = event-data() -> ("NewVal"=w326:bool)  [unwired: 1 in]
        n205 = case shown="False" w326 {
          tunnel: w325 -> [w335 _]
          tunnel: [w328 w346] -> w324
          tunnel: w323 -> [w327 w346]
          frame False {
            w342 = "Camera"
            w345 = FALSE ("Visible")
            n206 = local read "Camera Settings"() -> (w334:T3)
            n207 = Index Array(array=w335) -> (element=w338:cluster{string[]})  [unwired: 1 in]
            n208 = Unbundle(w334) -> ("Frame Rate"=w333:i32, "Compression"=w332:i32, "Size"=w336:u16)
            n209 = Unbundle(w338) -> (w337:string[])
            n210 = Index Array(array=w337, index=w336) -> (element=w331:string)
            n211 = call-poly <vilib>:"Write Key.vi"("section"=w342, "value"=w331, "key"="Size", "refnum"=w327) -> ("refnum out"=w344:T13)  [unwired: 2 in, 5 out]
            n212 = call-poly <vilib>:"Write Key.vi"("section"=w342, "value"=w333, "key"="FrameRate", "refnum"=w344) -> ("refnum out"=w343:T13)  [unwired: 1 in, 6 out]
            n213 = property on="Camera Settings" class="Clust (strict)"("Visible"=w345) -> ()  [unwired: 2 in, 2 out]
            n214 = local write "DB Camera Config"(w345) -> ()
            n215 = call-poly <vilib>:"Write Key.vi"("section"=w342, "value"=w332, "key"="Compression", "refnum"=w343) -> ("refnum out"=w329:T13)  [unwired: 1 in, 6 out]
            n216 = call <vilib>:"Close Config Data.vi"("refnum"=w329) -> ("file path"=w330:path)  [unwired: 2 in, 8 out]
            n217 = call <vilib>:"Open Config Data.vi"("configuration file path"=w330) -> ("refnum"=w328:T13)  [unwired: 8 in, 2 out]
          }
          frame True {
            n218 = property on="Camera Settings" class="Clust (strict)"("Visible"=TRUE) -> ()  [unwired: 2 in, 2 out]
          }
        }
      }
      event "Camera Settings": Value Change {
        n219 = event-data() -> ("NewVal"=w359:T3)  [unwired: 1 in]
        n220 = Index Array(array=w355) -> (element=w354:cluster{string[]})  [unwired: 1 in]
        n221 = Unbundle(w359) -> ("Frame Rate"=w350:i32, "Compression"=w349:i32, "Size"=w352:u16)
        n222 = Unbundle(w354) -> (w353:string[])
        n223 = Index Array(array=w353, index=w352) -> (element=w351:string)
        n224 = Format Into String(format string="%s   %dfps   %d%%", w351, w350, w349) -> (resulting string=w356:string)  [unwired: 2 in, 1 out]
        n225 = Build Array(w356) -> (w357:string[])
        n226 = property on="DB Camera Config" class="Bool (strict)"("Strings [4]"=w357) -> ()  [unwired: 2 in, 2 out]
      }
      event "Motor.Enable": Value Change {
        n227 = event-data() -> ("NewVal"=w365:bool)  [unwired: 1 in]
        n228 = Unbundle("Motor") -> ("Value"=w364:dbl)  [unwired: 1 out]
        n229 = Select(t=w364, s=w365, f=0.0) -> (s? t:f=w362:dbl)
        n230 = call <vilib>:"NT Write Number.vi"("Numeric"=w362, "Name"=w361) -> ()  [unwired: 9 in, 1 out]
      }
      event "Test Slider": Value Change {
        n231 = event-data() -> ("NewVal"=w368:dbl)  [unwired: 1 in]
        n232 = call <vilib>:"NT Write Number.vi"("Numeric"=w368, "Name"=w369) -> ()  [unwired: 9 in, 1 out]
      }
      event "On/Off": Value Change {
        n233 = event-data() -> ("NewVal"=w373:bool)  [unwired: 1 in]
        n234 = Boolean To (0,1)(Boolean=w373) -> (0, 1=w372:i16)
        n235 = call <vilib>:"NT Write Number.vi"("Numeric"=w372, "Name"=w371) -> ()  [unwired: 9 in, 1 out]
      }
      event "Rev/Fwd": Value Change {
        n236 = event-data() -> ("NewVal.Forward"=w381:bool, "NewVal.Reverse"=w380:bool)  [unwired: 1 in]
        n237 = Boolean To (0,1)(Boolean=w381) -> (0, 1=w377:i16)
        n238 = Boolean To (0,1)(Boolean=w380) -> (0, 1=w379:i16)
        n239 = Negate(x=w379) -> (-x=w378:i16)
        n240 = Add(x=w377, y=w378) -> (x+y=w376:i16)
        n241 = call <vilib>:"NT Write Number.vi"("Numeric"=w376, "Name"=w375) -> ()  [unwired: 9 in, 1 out]
      }
      event "Test Ring": Value Change {
        n242 = event-data() -> ("NewVal"=w385:u16)  [unwired: 1 in]
        n243 = property on="Test Ring" class="Ring (strict)"() -> ("Strings []"=w386:string[])  [unwired: 2 in, 2 out]
        n244 = Index Array(array=w386, index=w385) -> (element=w384:string)
        n245 = call <vilib>:"NT Write String.vi"("String"=w384, "Name"=w383) -> ()  [unwired: 9 in, 1 out]
      }
      event "Rec Mode": Value Change {
        # "Update globals for recording mode and path to read log from.\nClear when logging and let NetworkTables set path for vision to\nuse."
        n246 = event-data() -> ("NewVal"=w396:enum32{"Stop", "Record", "Playback"})  [unwired: 1 in]
        n247 = global write "WPI_DashboardLogging Global.vi" "Logging Filename"(path "") -> ()
        n248 = case shown="\"Stop\", \"Record\"" w396 {
          tunnel: w395 -> [_ w398 w406]
          tunnel: [_ _ w405] -> w392
          tunnel: [_ _ w404] -> _
          tunnel: w390 -> [_ _ w402]
          tunnel: cluster{i32, i32} {-250, 170} -> [_ _ w401]
          tunnel: [_ _ T15 {"Image Size"=TRUE, "Image Type"=TRUE, "Pixel Value"=TRUE, "ROI Information"=TRUE, "Zoom Factor"=FALSE} ("Image Information Shown:All Elements")] -> w388
          tunnel: [_ _ TRUE ("Zoom Factor")] -> w387
          frame Default {
          }
          frame "Stop", "Record" {
            # "Place Window too"
            n249 = invoke class="VI" method="FP.Close"(reference=w398) -> (reference out=w397:refnum<vi>)  [unwired: 2 in, 2 out]
            n250 = invoke class="VI" method="Abort VI"(reference=w397) -> ()  [unwired: 2 in, 3 out]
          }
          frame "Playback" {
            n251 = call "Open Playback Panel.vi"("Offset"=w401, "DB VI Ref"=w402, "Playback in"=w406) -> ("Playback out"=w403:refnum<vi>)  [unwired: 8 in]
            n252 = register-events(w403) -> (reference out=w405:refnum<event-registration>, error out=w404:errorcluster)  [unwired: 2 in]
          }
        }
        n253 = global write "WPI_DashboardLogging Global.vi" "Recording"(w396) -> ()
        n254 = property on="Camera Image" class="ImageControl"("Image Information Shown"=w388, "Image Information Visible"=w387) -> ()  [unwired: 2 in, 2 out]
        n255 = call <vilib>:"WPI_DashboardNT Log FieldName Cache.vi"("Operation"=enum16{"Lookup/Add", "Index", "Clear"}."Clear") -> ()  [unwired: 8 in, 3 out]
      }
      event Panel Close {
        w407 = enum32{"Stop", "Record", "Playback"}."Stop" ("Rec Mode")
        n256 = event-data() -> ()  [unwired: 1 in, 4 out]
        n257 = local write "Rec Mode"(w407) -> ()
        n258 = global write "WPI_DashboardLogging Global.vi" "Recording"(w407) -> ()
      }
      event Panel Close {
        # "Abort playback window and ourself"
        n259 = event-data() -> ()  [unwired: 1 in, 4 out]
        n260 = invoke class="VI" method="FP.Close"(reference=w412) -> (reference out=w411:refnum<vi>)  [unwired: 2 in, 2 out]
        n261 = invoke class="VI" method="Abort VI"(reference=w411) -> (error out=w410:errorcluster)  [unwired: 2 in, 2 out]
        n262 = invoke class="VI" method="Abort VI"(error in=w410) -> ()  [unwired: 2 in, 3 out]
      }
    }
  }
  n263 = property on="On/Off" class="Bool (strict)"("Visible"=w32) -> ()  [unwired: 2 in, 2 out]
  n264 = property on="Motor" class="Clust (strict)"("Visible"=w32) -> ()  [unwired: 2 in, 2 out]
  n265 = property on="Progress" class="Clust (strict)"("Visible"=w32) -> ()  [unwired: 2 in, 2 out]
  n266 = property on="Test Ring" class="Ring (strict)"("Visible"=w32) -> ()  [unwired: 2 in, 2 out]
  n267 = property on="Rev/Fwd" class="Clust (strict)"("Visible"=w32) -> ()  [unwired: 2 in, 2 out]
  n268 = property on="Camera Settings" class="Clust (strict)"("Visible"=w32) -> ()  [unwired: 2 in, 2 out]
  n269 = local write "DB Camera Config"(w32) -> ()
  n270 = global write "WPI_DashboardLogging Global.vi" "Recording"(w15) -> ()
  n271 = local write "Rec Mode"(w15) -> ()
  n272 = call "IMAQ Create"("Image Name"="Host Camera Image 2", "Image Type"=w5) -> ("New Image"=w3:T1)  [unwired: 2 in, 2 out]
  n273 = while {
    tunnel: w3 -> [w420]
    tunnel: [w421] -> _
    tunnel: "Camera Settings" -> [w414]
    tunnel: "Enable" -> [w413]
    i -> [w421]
    stop <- FALSE stop-if-true
    # "Optionally read the DB image,\nlog, or retrieve images from a\nlogged match"
    n274 = call <vilib>:"WPI_CameraRead MJPG for Dashboard.vi"("Camera Settings"=w414, "Camera IP"="10.1.78.12", "Enable"=w413, "Refnum in"=w420) -> ("Active"=w418:bool, "Refnum out"=w419:T1, "FPS"=w417:dbl, "Bandwidth (Mbps)"=w416:dbl)  [unwired: 4 in]
    n275 = case shown="True" w418 {
      tunnel: w419 -> [_ w425]
      tunnel: w416 -> [_ _]
      tunnel: w417 -> [_ _]
      frame False {
        # "Sleep for 500ms"
        n276 = Wait Until Next ms Multiple(millisecond multiple=u32 500) -> ()  [unwired: 1 out]
      }
      frame True {
        n277 = call "IMAQ Clear Overlay"("Image"=w425) -> ("Image Out"=→"Camera Image 2":T1)  [unwired: 2 in, 8 out]
      }
    }
  }
